vi "OLD MA3_Analog_Encoder.vi"(1 "s":bool, 2 "Sim":dbl, 3 "Elevator Encoder Ref":string="Elevator Encoder") -> (0 "Output":dbl)   [LabVIEW 2012]
panel:
  out "Numeric":dbl
  out "Code Output":dbl(graph)
  in  "Zero Encoder":dbl(slide)=-0.050505050505050594 scale=-5.0..5.0
  out "Offset":dbl
  out "Last":dbl(knob) scale=0.0..4.98
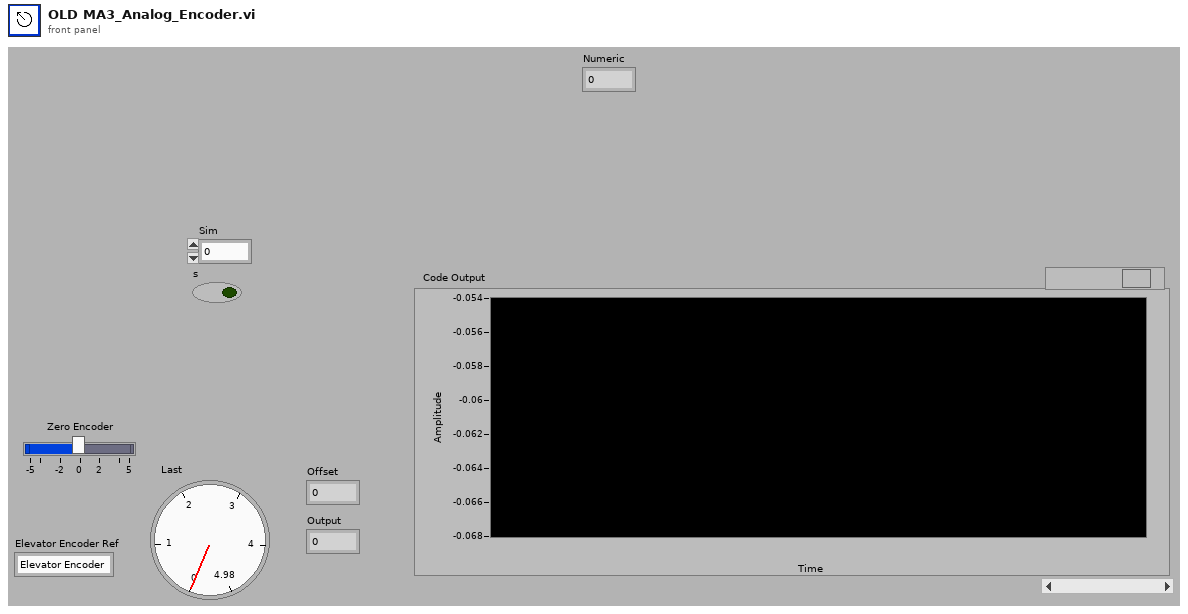
[diagram p1: front panel]
types:
  T1 = typedef "WPI_AnalogChannelDevRef.ctl" = cluster{"DevStatus":errorcluster, "Analog Module":T2, "Analog Channel":T3}
  T2 = typedef "FPGA_TypedefAnalogModule.ctl" = enum16{"Analog Module 1", "Analog Module 2"}
  T3 = typedef "FPGA_AIChannel.ctl" = enum8{"AI 1", "AI 2", "AI 3", "AI 4", "AI 5", "AI 6", "AI 7", "AI 8", "Invalid"}
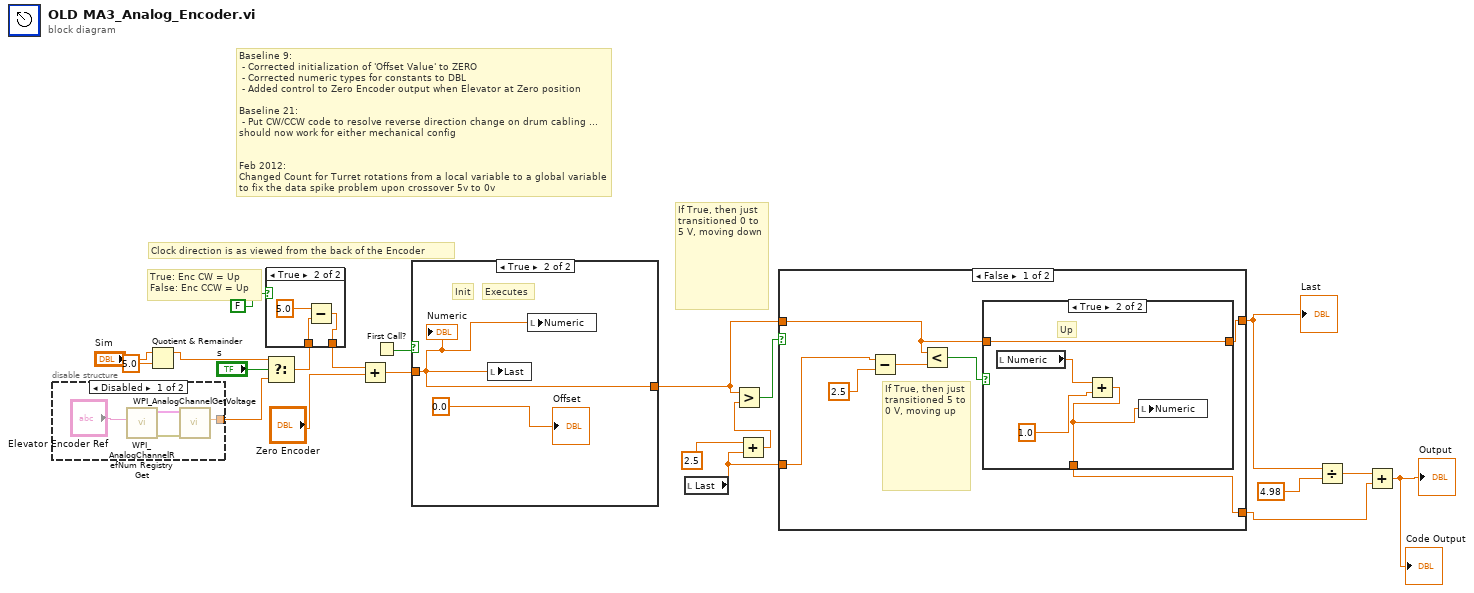
[diagram p0: block diagram]
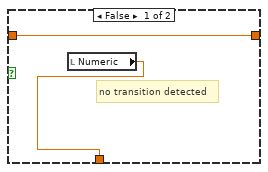
[diagram p4: hidden frame]
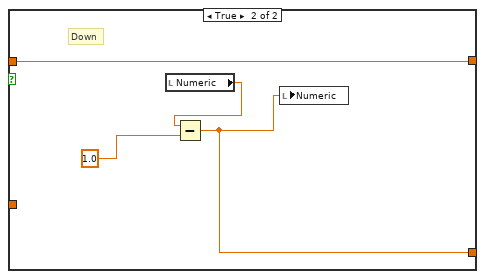
[diagram p5: hidden frame]
diagram:
  # "Clock direction is as viewed from the back of the Encoder"
  # "True: Enc CW = Up\nFalse: Enc CCW = Up"
  # "Baseline 9:\n - Corrected initialization of 'Offset Value' to ZERO\n - Corrected numeric types for constants to DBL\n - Added control to Zero Encoder output when Elevator at Zero position\n\nBaseline 21:\n - Put CW/CCW code to resolve reverse direction change on drum cabling ... should now work for either mechanical config\n \n\nFeb 2012:\nChanged Count for Turret rotations from a local variable to a global variable to fix the data spike problem upon crossover 5v to 0v"
  # "If True, then just transitioned 0 to 5 V, moving down"
  n1 = disable-structure shown="Disabled" {
    disable-tunnel: [w22 _] -> w5
    frame Disabled {
      n2 = call <vilib>:"WPI_AnalogChannelRefNum Registry Get.vi"("refnum name"="Elevator Encoder Ref") -> ("error out"=w24:errorcluster, "AIDeviceRef"=w25:T1)  [unwired: 1 in, 8 out]
      n3 = call <vilib>:"WPI_AnalogChannelGetVoltage.vi"("error in (no error)"=w24, "AIDeviceRef"=w25) -> ("Voltage"=w22:dbl)  [unwired: 9 out]
    }
    frame Enabled {
    }
  }
  n4 = Quotient & Remainder(x="Sim", y=5.0) -> (x-y*floor(x/y)=w2:dbl)  [unwired: 1 out]
  n5 = Select(t=w2, s="s", f=w5) -> (s? t:f=w6:dbl)
  n6 = case shown="True" FALSE {
    tunnel: w6 -> [w26 w28]
    tunnel: [w26 w27] -> w10
    frame False {
    }
    frame True {
      n7 = Subtract(x=5.0, y=w28) -> (x-y=w27:dbl)
    }
  }
  n8 = Add(x=w10, y="Zero Encoder") -> (x+y=w9:dbl)
  n9 = First Call?() -> (First Call?: T/F=w13:bool)
  n10 = case shown="True" w13 {
    tunnel: w9 -> [w30 w31]
    tunnel: [w30 w31] -> w17
    frame False {
    }
    frame True {
      # "Executes"
      # "Init"
      n11 = local write "Last"(w31) -> ()
      n12 = local write "Numeric"(w31) -> ()
      "Offset" <- 0.0
      "Numeric" <- w31
    }
  }
  n13 = local read "Last"() -> (w18:dbl)
  n14 = Add(x=2.5, y=w18) -> (x+y=w20:dbl)
  n15 = Greater?(x=w17, y=w20) -> (0:w19:bool)
  n16 = case shown="False" w19 {
    tunnel: w18 -> [w36 _]
    tunnel: w17 -> [w35 w48]
    tunnel: [w34 w48] -> w14
    tunnel: [w33 w46] -> w7
    frame False {
      # "If True, then just transitioned 5 to 0 V, moving up"
      n17 = Subtract(x=w36, y=2.5 ("x")) -> (x-y=w38:dbl)
      n18 = Less?(x=w35, y=w38) -> (x < y?=w37:bool)
      n19 = case shown="True" w37 {
        tunnel: [w41 w45] -> w34
        tunnel: w35 -> [w41 w45]
        tunnel: [w40 w43] -> w33
        frame False {
          # "no transition detected"
          n20 = local read "Numeric"() -> (w40:dbl)
        }
        frame True {
          # "Up"
          n21 = local read "Numeric"() -> (w42:dbl)
          n22 = Add(x=w42, y=1.0) -> (x+y=w43:dbl)
          n23 = local write "Numeric"(w43) -> ()
        }
      }
    }
    frame True {
      # "Down"
      n24 = local read "Numeric"() -> (w47:dbl)
      n25 = Subtract(x=w47, y=1.0) -> (x-y=w46:dbl)
      n26 = local write "Numeric"(w46) -> ()
    }
  }
  "Last" <- w14
  n27 = Divide(x=w14, y=4.98) -> (x/y=w16:dbl)
  n28 = Add(x=w16, y=w7) -> (x+y=→"Output" →"Code Output":dbl)
